vi "Client Test.vi"() -> ()   [LabVIEW 2018, in "OPC UA.lvlib"]
uses:
  OPC UA.lvlib
  Object Data Array Cluster.ctl
  Object Data Cluster.ctl
  Variable Data Cluster.ctl
  <vilib>/OPCUA/controls/NodeId.ctl
  <vilib>/OPCUA/controls/OPC UA StatusCode.ctl
  <vilib>/OPCUA/controls/NodeIds.ctl
  <vilib>/OPCUA/controls/Write Variant Request.ctl
  <vilib>/OPCUA/controls/Write Status.ctl
  support/Message Queue/Enqueue Message (Single).vi
  <vilib>/OPCUA/client/Multiple Write Variant.vi
  <vilib>/OPCUA/NI OPC UA Client.lvlib
  support/Message Queue/Message Queue.lvlib
panel:
  out "Object Cluster":T1
  in  "Numeric":dbl
  in  "Send":bool
  in  "Variable Ring":u16(ring) items=["Default", "TestVariable1", "TestVariable2", "TestVariable3"]
  in  "Object Ring":u16(ring) items=["Default"]
  in  "security policy":T2
  in  "stop":bool
  out "Waveform Chart":i32(graph)
  out "OPC Server Data":T3 {"Variable Array"."status" items=["Good"=0, "Good_SubscriptionTransferred"=2949120, "Good_CompletesAsynchronously"=3014656, "Good_Overload"=3080192, "Good_Clamped"=3145728, "Good_LocalOverride"=9830400, "Good_EntryInserted"=10616832, "Good_EntryReplaced"=10682368, "Good_NoData"=10813440, "Good_MoreData"=10878976, "Good_CommunicationEvent"=10944512, "Good_ShutdownEvent"=11010048, "Good_CallAgain"=11075584, "Good_NonCriticalTimeout"=11141120, "Good_ResultsMayBeIncomplete"=12189696, "Good_DataIgnored"=14221312, "Uncertain"=1073741824, "Uncertain_ReferenceOutOfServer"=1080819712, "Uncertain_NoCommunicationLastUsableValue"=1083113472, "Uncertain_LastUsableValue"=1083179008, "Uncertain_SubstituteValue"=1083244544, "Uncertain_InitialValue"=1083310080, "Uncertain_SensorNotAccurate"=1083375616, "Uncertain_EngineeringUnitsExceeded"=1083441152, "Uncertain_SubNormal"=1083506688, "Uncertain_DataSubNormal"=1084489728, "Uncertain_ReferenceNotDeleted"=1086062592, "Uncertain_NotAllNodesAvailable"=1086324736, "Bad"=2147483648, "Bad_UnexpectedError"=2147549184, "Bad_InternalError"=2147614720, "Bad_OutOfMemory"=2147680256, "Bad_ResourceUnavailable"=2147745792, "Bad_CommunicationError"=2147811328, "Bad_EncodingError"=2147876864, "Bad_DecodingError"=2147942400, "Bad_EncodingLimitsExceeded"=2148007936, "Bad_UnknownResponse"=2148073472, "Bad_Timeout"=2148139008, "Bad_ServiceUnsupported"=2148204544, "Bad_Shutdown"=2148270080, "Bad_ServerNotConnected"=2148335616, "Bad_ServerHalted"=2148401152, "Bad_NothingToDo"=2148466688, "Bad_TooManyOperations"=2148532224, "Bad_DataTypeIdUnknown"=2148597760, "Bad_CertificateInvalid"=2148663296, "Bad_SecurityChecksFailed"=2148728832, "Bad_CertificateTimeInvalid"=2148794368, "Bad_CertificateIssuerTimeInvalid"=2148859904, "Bad_CertificateHostNameInvalid"=2148925440, "Bad_CertificateUriInvalid"=2148990976, "Bad_CertificateUseNotAllowed"=2149056512, "Bad_CertificateIssuerUseNotAllowed"=2149122048, "Bad_CertificateUntrusted"=2149187584, "Bad_CertificateRevocationUnknown"=2149253120, "Bad_CertificateIssuerRevocationUnknown"=2149318656, "Bad_CertificateRevoked"=2149384192, "Bad_CertificateIssuerRevoked"=2149449728, "Bad_UserAccessDenied"=2149515264, "Bad_IdentityTokenInvalid"=2149580800, "Bad_IdentityTokenRejected"=2149646336, "Bad_SecureChannelIdInvalid"=2149711872, "Bad_InvalidTimestamp"=2149777408, "Bad_NonceInvalid"=2149842944, "Bad_SessionIdInvalid"=2149908480, "Bad_SessionClosed"=2149974016, "Bad_SessionNotActivated"=2150039552, "Bad_SubscriptionIdInvalid"=2150105088, "Bad_RequestHeaderInvalid"=2150236160, "Bad_TimestampsToReturnInvalid"=2150301696, "Bad_RequestCancelledByClient"=2150367232, "Bad_NoCommunication"=2150694912, "Bad_WaitingForInitialData"=2150760448, "Bad_NodeIdInvalid"=2150825984, "Bad_NodeIdUnknown"=2150891520, "Bad_AttributeIdInvalid"=2150957056, "Bad_IndexRangeInvalid"=2151022592, "Bad_IndexRangeNoData"=2151088128, "Bad_DataEncodingInvalid"=2151153664, "Bad_DataEncodingUnsupported"=2151219200, "Bad_NotReadable"=2151284736, "Bad_NotWritable"=2151350272, "Bad_OutOfRange"=2151415808, "Bad_NotSupported"=2151481344, "Bad_NotFound"=2151546880, "Bad_ObjectDeleted"=2151612416, "Bad_NotImplemented"=2151677952, "Bad_MonitoringModeInvalid"=2151743488, "Bad_MonitoredItemIdInvalid"=2151809024, "Bad_MonitoredItemFilterInvalid"=2151874560, "Bad_MonitoredItemFilterUnsupported"=2151940096, "Bad_FilterNotAllowed"=2152005632, "Bad_StructureMissing"=2152071168, "Bad_EventFilterInvalid"=2152136704, "Bad_ContentFilterInvalid"=2152202240, "Bad_FilterOperandInvalid"=2152267776, "Bad_ContinuationPointInvalid"=2152333312, "Bad_NoContinuationPoints"=2152398848, "Bad_ReferenceTypeIdInvalid"=2152464384, "Bad_BrowseDirectionInvalid"=2152529920, "Bad_NodeNotInView"=2152595456, "Bad_ServerUriInvalid"=2152660992, "Bad_ServerNameMissing"=2152726528, "Bad_DiscoveryUrlMissing"=2152792064, "Bad_SempahoreFileMissing"=2152857600, "Bad_RequestTypeInvalid"=2152923136, "Bad_SecurityModeRejected"=2152988672, "Bad_SecurityPolicyRejected"=2153054208, "Bad_TooManySessions"=2153119744, "Bad_UserSignatureInvalid"=2153185280, "Bad_ApplicationSignatureInvalid"=2153250816, "Bad_NoValidCertificates"=2153316352, "Bad_RequestCancelledByRequest"=2153381888, "Bad_ParentNodeIdInvalid"=2153447424, "Bad_ReferenceNotAllowed"=2153512960, "Bad_NodeIdRejected"=2153578496, "Bad_NodeIdExists"=2153644032, "Bad_NodeClassInvalid"=2153709568, "Bad_BrowseNameInvalid"=2153775104, "Bad_BrowseNameDuplicated"=2153840640, "Bad_NodeAttributesInvalid"=2153906176, "Bad_TypeDefinitionInvalid"=2153971712, "Bad_SourceNodeIdInvalid"=2154037248, "Bad_TargetNodeIdInvalid"=2154102784, "Bad_DuplicateReferenceNotAllowed"=2154168320, "Bad_InvalidSelfReference"=2154233856, "Bad_ReferenceLocalOnly"=2154299392, "Bad_NoDeleteRights"=2154364928, "Bad_ServerIndexInvalid"=2154430464, "Bad_ViewIdUnknown"=2154496000, "Bad_TooManyMatches"=2154627072, "Bad_QueryTooComplex"=2154692608, "Bad_NoMatch"=2154758144, "Bad_MaxAgeInvalid"=2154823680, "Bad_HistoryOperationInvalid"=2154889216, "Bad_HistoryOperationUnsupported"=2154954752, "Bad_WriteNotSupported"=2155020288, "Bad_TypeMismatch"=2155085824, "Bad_MethodInvalid"=2155151360, "Bad_ArgumentsMissing"=2155216896, "Bad_TooManySubscriptions"=2155282432, "Bad_TooManyPublishRequests"=2155347968, "Bad_NoSubscription"=2155413504, "Bad_SequenceNumberUnknown"=2155479040, "Bad_MessageNotAvailable"=2155544576, "Bad_InsufficientClientProfile"=2155610112, "Bad_TcpServerTooBusy"=2155675648, "Bad_TcpMessageTypeInvalid"=2155741184, "Bad_TcpSecureChannelUnknown"=2155806720, "Bad_TcpMessageTooLarge"=2155872256, "Bad_TcpNotEnoughResources"=2155937792, "Bad_TcpInternalError"=2156003328, "Bad_TcpEndpointUrlInvalid"=2156068864, "Bad_RequestInterrupted"=2156134400, "Bad_RequestTimeout"=2156199936, "Bad_SecureChannelClosed"=2156265472, "Bad_SecureChannelTokenUnknown"=2156331008, "Bad_SequenceNumberInvalid"=2156396544, "Bad_ConfigurationError"=2156462080, "Bad_NotConnected"=2156527616, "Bad_DeviceFailure"=2156593152, "Bad_SensorFailure"=2156658688, "Bad_OutOfService"=2156724224, "Bad_DeadbandFilterInvalid"=2156789760, "Bad_RefreshInProgress"=2157379584, "Bad_ConditionAlreadyDisabled"=2157445120, "Bad_ConditionDisabled"=2157510656, "Bad_EventIdUnknown"=2157576192, "Bad_NoData"=2157641728, "Bad_DataLost"=2157772800, "Bad_DataUnavailable"=2157838336, "Bad_EntryExists"=2157903872, "Bad_NoEntryExists"=2157969408, "Bad_TimestampNotSupported"=2158034944, "Bad_InvalidArgument"=2158690304, "Bad_ConnectionRejected"=2158755840, "Bad_Disconnect"=2158821376, "Bad_ConnectionClosed"=2158886912, "Bad_InvalidState"=2158952448, "Bad_EndOfStream"=2159017984, "Bad_NoDataAvailable"=2159083520, "Bad_WaitingForResponse"=2159149056, "Bad_OperationAbandoned"=2159214592, "Bad_ExpectedStreamToBlock"=2159280128, "Bad_WouldBlock"=2159345664, "Bad_SyntaxError"=2159411200, "Bad_MaxConnectionsReached"=2159476736, "Bad_RequestTooLarge"=2159542272, "Bad_ResponseTooLarge"=2159607808, "Bad_EventNotAcknowledgeable"=2159738880, "Bad_InvalidTimestampArgument"=2159869952, "Bad_ProtocolVersionUnsupported"=2159935488, "Bad_StateNotActive"=2160001024, "Bad_FilterOperatorInvalid"=2160132096, "Bad_FilterOperatorUnsupported"=2160197632, "Bad_FilterOperandCountMismatch"=2160263168, "Bad_FilterElementInvalid"=2160328704, "Bad_FilterLiteralInvalid"=2160394240, "Bad_IdentityChangeNotSupported"=2160459776, "Bad_NotTypeDefinition"=2160590848, "Bad_ViewTimestampInvalid"=2160656384, "Bad_ViewParameterMismatch"=2160721920, "Bad_ViewVersionInvalid"=2160787456, "Bad_ConditionAlreadyEnabled"=2160852992, "Bad_DialogNotActive"=2160918528, "Bad_DialogResponseInvalid"=2160984064, "Bad_ConditionBranchAlreadyAcked"=2161049600, "Bad_ConditionBranchAlreadyConfirmed"=2161115136, "Bad_ConditionAlreadyShelved"=2161180672, "Bad_ConditionNotShelved"=2161246208, "Bad_ShelvingTimeOutOfRange"=2161311744, "Bad_AggregateListMismatch"=2161377280, "Bad_AggregateNotSupported"=2161442816, "Bad_AggregateInvalidInputs"=2161508352, "Bad_BoundNotFound"=2161573888, "Bad_BoundNotSupported"=2161639424, "Bad_AggregateConfigurationRejected"=2161770496, "Bad_TooManyMonitoredItems"=2161836032]}
  in  "server endpoint URL":string="opc.tcp://10.131.1.22:4840"
  # "opc.tcp://10.131.1.22:4840"
  # "opc.tcp://127.0.0.1:49320"
  # "opc.tcp://AMRGROBJ07MYKD.amer.pfizer.com:49320"
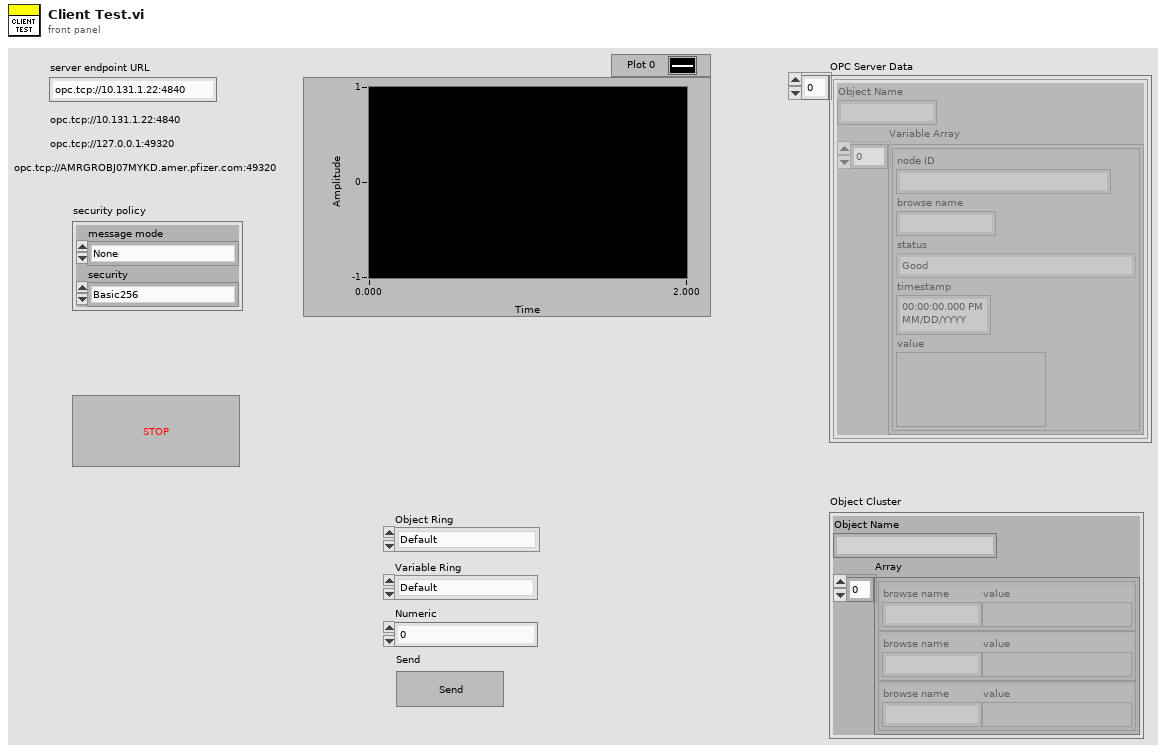
[diagram p1: front panel]
types:
  T1 = cluster{"Object Name":string, "Array":cluster{"browse name":string, "value ":variant}[]}
  T2 = cluster{"message mode":enum16{"None", "Sign", "Sign and Encrypt"}, "security":enum16{"Basic256", "Basic128Rsa15"}}
  T3 = typedef "OPC UA.lvlib/Object Data Array Cluster.ctl" = T4[]
  T4 = typedef "OPC UA.lvlib/Object Data Cluster.ctl" = cluster{"Object Name":string, "Variable Array":T5[]}
  T5 = typedef "OPC UA.lvlib/Variable Data Cluster.ctl" = cluster{"node ID":T6, "browse name":string, "status":T7, "timestamp":timestamp, "value ":variant}
  T6 = typedef "NodeId.ctl" = string
  T7 = typedef "OPC UA StatusCode.ctl" = u32
  T8 = typedef "NodeIds.ctl" = T6[]
  T9 = typedef "OPC UA Client Refnum.ctl" = refnum<k21>
  T10 = typedef "Subscription ID.ctl" = u32
  T11 = typedef "Write Variant Request.ctl" = cluster{"node ID":T6, "value":variant, "timestamp (current time)":timestamp, "node status":T12}
  T12 = typedef "Write Status.ctl" = u32
  T13 = typedef "Subscription Data Change.ctl" = cluster{"node ID":T6, " value":variant, "timestamp":timestamp, "data type":T14, "status code":T7}
  T14 = typedef "Data Type.ctl" = u16
  T15 = typedef "Node Class.ctl" = u32
  T16 = cluster{"reference type":u32, "node ID":T6, "browse name":string, "node class":T15, "node type":u32}[]
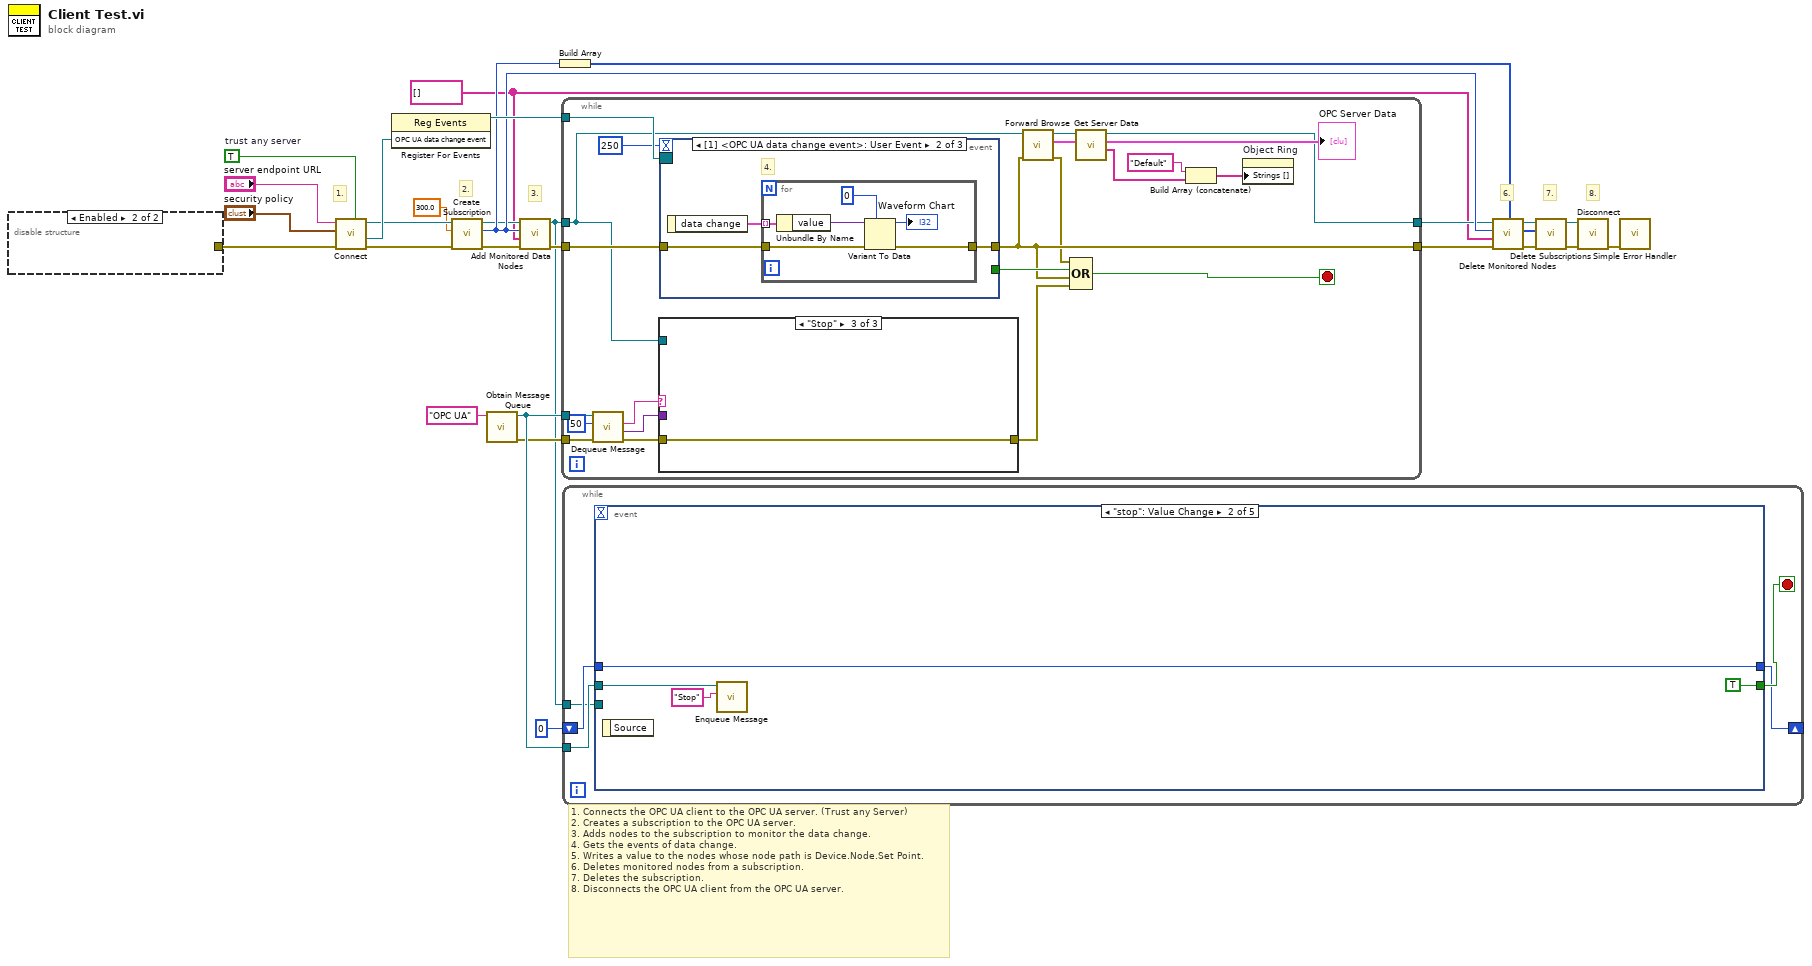
[diagram p0: block diagram]
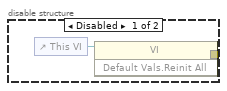
[diagram p2: hidden frame]
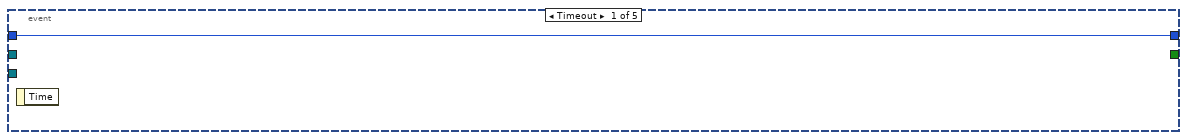
[diagram p3: hidden frame]
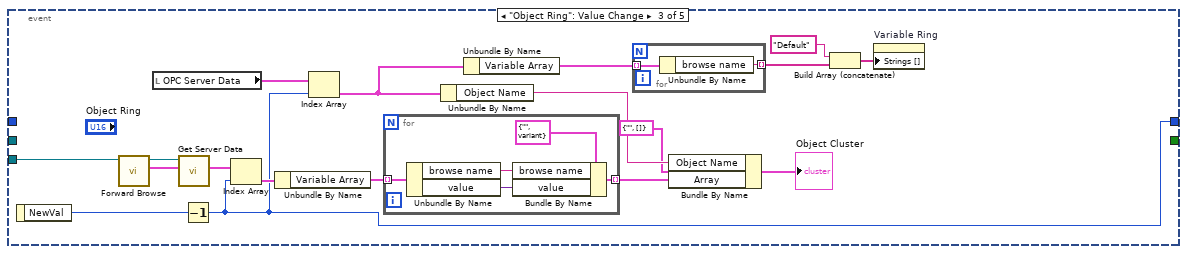
[diagram p4: hidden frame]
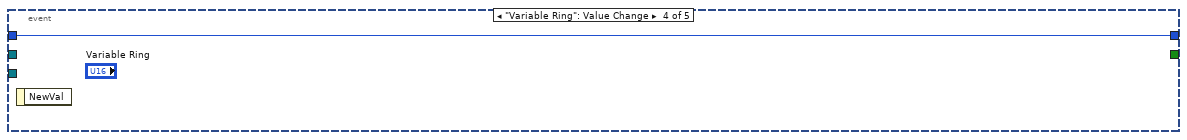
[diagram p5: hidden frame]
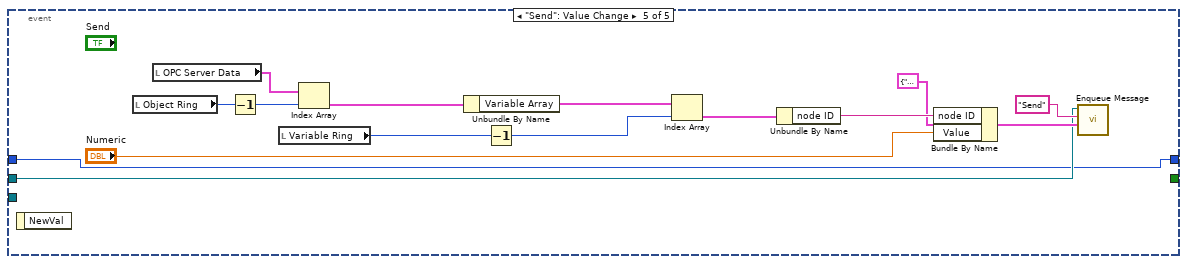
[diagram p6: hidden frame]
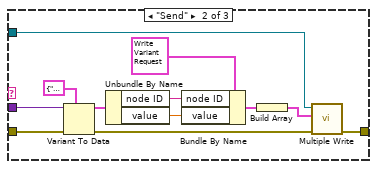
[diagram p8: hidden frame]
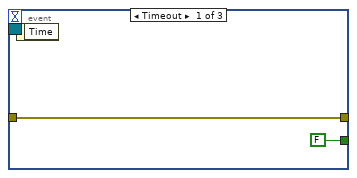
[diagram p9: hidden frame]
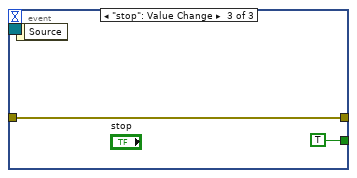
[diagram p10: hidden frame]
diagram:
  w4 = T8 [] ("node IDs")
  w11 = TRUE  # trust any server
  # "7."
  # "1. Connects the OPC UA client to the OPC UA server. (Trust any Server) \n2. Creates a subscription to the OPC UA server.\n3. Adds nodes to the subscription to monitor the data change.\n4. Gets the events of data change.\n5. Writes a value to the nodes whose node path is Device.Node.Set Point. \n6. Deletes monitored nodes from a subscription.\n7. Deletes the subscription.\n8. Disconnects the OPC UA client from the OPC UA server."
  # "8."
  # "6."
  # "3."
  # "2."
  # "1."
  n1 = disable-structure shown="Enabled" {
    disable-tunnel: [w28 _] -> w2
    frame Disabled {
      n2 = control-ref of="This VI"() -> (w29:refnum<vi>)
      n3 = invoke class="VI" method="Default Vals.Reinit All"(reference=w29) -> (error out=w28:errorcluster)  [unwired: 2 in, 2 out]
    }
    frame Enabled {
    }
  }
  n4 = call <vilib>:"Connect.vi"("trust any server (F)"=w11, "error in (no error)"=w2, "security policy"="security policy", "server endpoint URL"="server endpoint URL") -> ("error out"=w1:errorcluster, "OPC UA data change event"=w25:refnum<user-event>, "OPC UA client refnum out"=w17:T9)  [unwired: 5 in]
  n5 = register-events(w25) -> (reference out=w24:refnum<event-registration>)  [unwired: 2 in, 1 out]
  n6 = call <vilib>:"Create Subscription.vi"("error in (no error)"=w1, "publishing interval (1000 ms)"=300.0 ("update rate (1000 ms)"), "OPC UA client refnum in"=w17) -> ("error out"=w26:errorcluster, "subscription ID out"=w15:T10, "OPC UA client refnum out"=w10:T9)  [unwired: 4 in, 2 out]
  n7 = call "Obtain Message Queue.vi"("name (unnamed)"="OPC UA") -> ("error out"=w6:errorcluster, "Message Queue"=w7:refnum<queue>)  [unwired: 9 in]
  n8 = call <vilib>:"Add Monitored Data Nodes.vi"("error in (no error)"=w26, "node IDs"=w4, "subscription ID in"=w15, "OPC UA client refnum in"=w10) -> ("error out"=w23:errorcluster, "OPC UA client refnum out"=w3:T9)  [unwired: 4 in, 2 out]
  n9 = Build Array(w15) -> (w14:T10[])
  n10 = while {
    tunnel: w24 -> [w51]
    tunnel: w3 -> [w41]
    tunnel: w23 -> [w49]
    tunnel: [w31] -> w22
    tunnel: [w45] -> w9
    tunnel: w7 -> [w44]
    tunnel: w6 -> [w43]
    stop <- w33 stop-if-true
    n11 = call "Dequeue Message.vi"("error in (no error)"=w43, "timeout in ms (-1)"=50, "Message Queue"=w44) -> ("error out"=w39:errorcluster, "Message Data"=w40:variant, "Message"=w42:string)  [unwired: 5 in, 1 out]
    n12 = case shown="\"Stop\"" w42 {
      tunnel: w41 -> [_ w61 _]
      tunnel: w40 -> [_ w59 _]
      tunnel: w39 -> [w52 w60 w65]
      tunnel: [w52 w53 w65] -> w34
      frame "Timeout", Default {
      }
      frame "Send" {
        n13 = Variant To Data(error in=w60, type=cluster{"node ID":string, "value":dbl} {"node ID"="", "value"=0.0}, Variant=w59) -> (data=w57:cluster{"node ID":string, "value":dbl}, error out=w54:errorcluster)
        n14 = Unbundle By Name(w57) -> ("node ID"=w56:string, "value"=w55:dbl)
        n15 = Bundle By Name(cluster=T11 {"node ID"="ns=2;i=4", "value"=variant, "timestamp (current time)"=timestamp(0 s since 1904-01-01), "node status"=0} ("request"), "node ID"=w56, "value"=w55) -> (w62:T11)
        n16 = Build Array(w62) -> (w63:T11[])
        n17 = call-poly <vilib>:"Multiple Write.vi"("error in (no error)"=w54, "requests"=w63, "OPC UA client refnum in"=w61) -> ("error out"=w53:errorcluster)  [unwired: 5 in, 3 out]
      }
      frame "Stop" {
      }
    }
    n18 = event shown="[1] <OPC UA data change event>: User Event" {
      selector: w51 -> [_ _ _]
      dyn-events: _ -> [_ _ _]
      timeout: 250 -> [_ _ _]
      tunnel: [w67 w68 w77] -> w31
      tunnel: w49 -> [w67 w69 w77]
      tunnel: [FALSE _ TRUE] -> w32
      event Timeout {
        n19 = event-data() -> ()  [unwired: 1 in, 1 out]
      }
      event User Event {
        # "4."
        n20 = event-data() -> ("data change"=w70:T13[])  [unwired: 1 in]
        n21 = for {
          tunnel: w70 -> [w76] mode=indexing
          tunnel: w69 -> [w72]
          tunnel: [w71] -> w68
          n22 = Unbundle By Name(w76) -> ("value"=w75:variant)
          n23 = Variant To Data(error in=w72, type=0, Variant=w75) -> (data=→"Waveform Chart":i32, error out=w71:errorcluster)
        }
      }
      event "stop": Value Change {
        n24 = event-data() -> ()  [unwired: 1 in, 1 out]
      }
    }
    n25 = call <vilib>:"Forward Browse.vi"("error in (no error)"=w31, "OPC UA client refnum in"=w41) -> ("error out"=w30:errorcluster, "browse result"=w47:T16, "OPC UA client refnum out"=w48:T9)  [unwired: 6 in, 1 out]
    n26 = Compound Arithmetic op=OR(w30, w32, w31, w34) -> (w33:bool)
    n27 = call "Get Server Data.vi"("browse result"=w47, "OPC UA Client in"=w48) -> ("Browse Names"=w37:string[], "OPC Server Data"=→"OPC Server Data":T4[], "OPC UA Client Refnum out"=w45:T9)  [unwired: 7 in]
    n28 = Build Array (concatenate)("Default", w37) -> (w35:string[])
    n29 = property on="Object Ring" class="Ring (strict)"("Strings []"=w35) -> ()  [unwired: 2 in, 2 out]
  }
  n30 = while {
    shift-right: [w82] -> _
    shift-left: u16 0 ("NewVal") -> [w81]
    tunnel: w7 -> [w80]
    tunnel: w3 -> [w79]
    stop <- w83 stop-if-true
    n31 = event shown="[1] \"stop\": Value Change" {
      selector: _ -> [_ _ _ _ _]
      dyn-events: _ -> [_ _ _ _ _]
      timeout: _ -> [_ _ _ _ _]
      tunnel: [_ TRUE _ _ _] -> w83
      tunnel: [w84 w85 w89 w114 w119] -> w82
      tunnel: w81 -> [w84 w85 _ w114 w119]
      tunnel: w80 -> [_ w86 _ _ w120]
      tunnel: w79 -> [_ _ w96 _ _]
      event Timeout {
        n32 = event-data() -> ()  [unwired: 1 in, 1 out]
      }
      event "stop": Value Change {
        n33 = event-data() -> ()  [unwired: 1 in, 1 out]
        n34 = call-poly "Enqueue Message.vi"("Message"="Stop", "Message Queue"=w86) -> ()  [unwired: 8 in, 2 out]
      }
      event "Object Ring": Value Change {
        n35 = event-data() -> ("NewVal"=w102:u16)  [unwired: 1 in]
        n36 = call <vilib>:"Forward Browse.vi"("OPC UA client refnum in"=w96) -> ("browse result"=w94:T16, "OPC UA client refnum out"=w95:T9)  [unwired: 7 in, 2 out]
        n37 = local read "OPC Server Data"() -> (w106:T3)
        n38 = call "Get Server Data.vi"("browse result"=w94, "OPC UA Client in"=w95) -> ("OPC Server Data"=w92:T4[])  [unwired: 7 in, 2 out]
        n39 = Decrement(x=w102) -> (x-1=w89:u16)
        n40 = Index Array(array=w92, index=w89) -> (element=w91:T4)
        n41 = Unbundle By Name(w91) -> ("Variable Array"=w93:T5[])
        n42 = Index Array(array=w106, index=w89) -> (element=w101:T4)
        n43 = for {
          tunnel: w93 -> [w111] mode=indexing
          tunnel: [w107] -> w90 mode=indexing
          n44 = Unbundle By Name(w111) -> ("browse name"=w109:string, "value"=w108:variant)
          n45 = Bundle By Name(cluster=cluster{"browse name":string, "value ":variant} {"browse name"="", "value "=variant} ("Object Data"), "browse name"=w109, "value"=w108) -> (w107:cluster{"browse name":string, "value ":variant})
        }
        n46 = Unbundle By Name(w101) -> ("Object Name"=w100:string)
        n47 = Unbundle By Name(w101) -> ("Variable Array"=w105:T5[])
        n48 = for {
          tunnel: w105 -> [w113] mode=indexing
          tunnel: [w112] -> w103 mode=indexing
          n49 = Unbundle By Name(w113) -> ("browse name"=w112:string)
        }
        n50 = Bundle By Name(cluster=T1 {"Object Name"="", "Array"=[]} ("Object Cluster"), "Object Name"=w100, "Array"=w90) -> (→"Object Cluster":T1)
        n51 = Build Array (concatenate)("Default", w103) -> (w99:string[])
        n52 = property on="Variable Ring" class="Ring (strict)"("Strings []"=w99) -> ()  [unwired: 2 in, 2 out]
      }
      event "Variable Ring": Value Change {
        n53 = event-data() -> ()  [unwired: 1 in, 1 out]
      }
      event "Send": Value Change {
        n54 = event-data() -> ()  [unwired: 1 in, 1 out]
        n55 = local read "Object Ring"() -> (w118:u16)
        n56 = local read "OPC Server Data"() -> (w123:T3)
        n57 = Decrement(x=w118) -> (x-1=w117:u16)
        n58 = local read "Variable Ring"() -> (w116:u16)
        n59 = Index Array(array=w123, index=w117) -> (element=w124:T4)
        n60 = Unbundle By Name(w124) -> ("Variable Array"=w125:T5[])
        n61 = Decrement(x=w116) -> (x-1=w115:u16)
        n62 = Index Array(array=w125, index=w115) -> (element=w126:T5)
        n63 = Unbundle By Name(w126) -> ("node ID"=w127:T6)
        n64 = Bundle By Name(cluster=cluster{"node ID":string, "Value":dbl} {"node ID"="", "Value"=0.0}, "node ID"=w127, "Value"="Numeric") -> (w129:cluster{"node ID":string, "Value":dbl})
        n65 = call-poly "Enqueue Message.vi"("Message Data"=w129, "Message"="Send", "Message Queue"=w120) -> ()  [unwired: 7 in, 2 out]
      }
    }
  }
  n66 = call <vilib>:"Delete Monitored Nodes.vi"("error in (no error)"=w22, "node IDs"=w4, "subscription ID in"=w15, "OPC UA client refnum in"=w9) -> ("error out"=w20:errorcluster, "OPC UA client refnum out"=w21:T9)  [unwired: 3 in, 3 out]
  n67 = call <vilib>:"Delete Subscriptions.vi"("error in (no error)"=w20, "subscription IDs"=w14, "OPC UA client refnum in"=w21) -> ("error out"=w18:errorcluster, "OPC UA client refnum out"=w19:T9)  [unwired: 6 in, 1 out]
  n68 = call <vilib>:"Disconnect.vi"("error in (no error)"=w18, "OPC UA client refnum in"=w19) -> ("error out"=w12:errorcluster)  [unwired: 9 in]
  n69 = call <vilib>:"Simple Error Handler.vi"("error in (no error)"=w12) -> ()  [unwired: 4 in, 5 out]
